vi "worker_loop.vi"(8 "error in (no error)":errorcluster, 10 "Notifiers":T1, 11 "Message Queues":T2) -> (0 "error out":errorcluster)   [LabVIEW 2017, in "worker.lvlib"]
uses:
  worker.lvlib
  support/Message Queue/All Message Queues.ctl
  support/Message Queue/Message Cluster.ctl
  support/Notifiers/Notifiers.ctl
  support/my_global.vi
  <vilib>/Utility/error.llb/Error Cluster From Error Code.vi
  <vilib>/ErrorRing/Error Ring.xnode
  support/Message Queue/Message Queue.lvlib
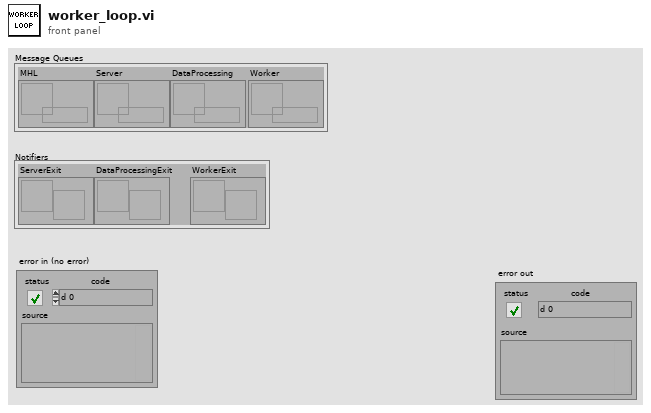
[diagram p1: front panel]
types:
  T1 = typedef "Notifiers.ctl" = cluster{"ServerExit":refnum<notifier>, "DataProcessingExit":refnum<notifier>, "WorkerExit":refnum<notifier>}
  T2 = typedef "Message Queue.lvlib/All Message Queues.ctl" = cluster{"MHL":refnum<queue>, "Server":refnum<queue>, "DataProcessing":refnum<queue>, "Worker":refnum<queue>}
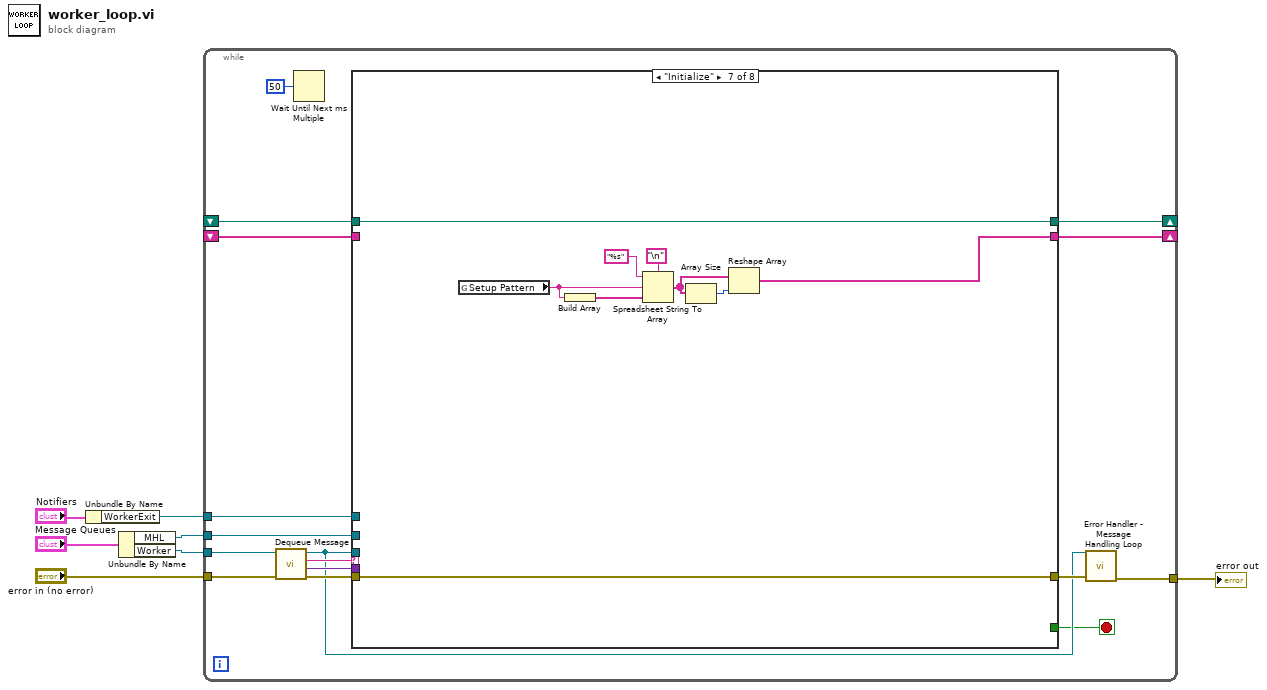
[diagram p0: block diagram]
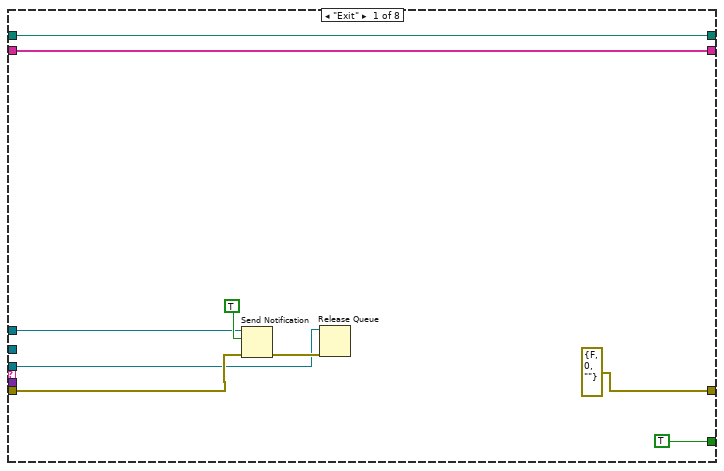
[diagram p2: hidden frame]
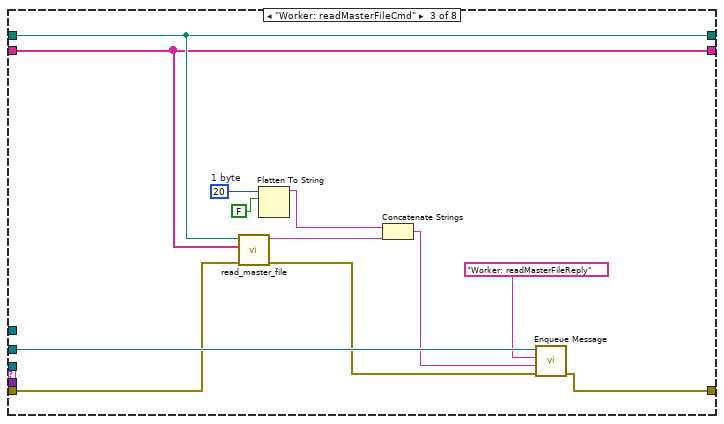
[diagram p4: hidden frame]
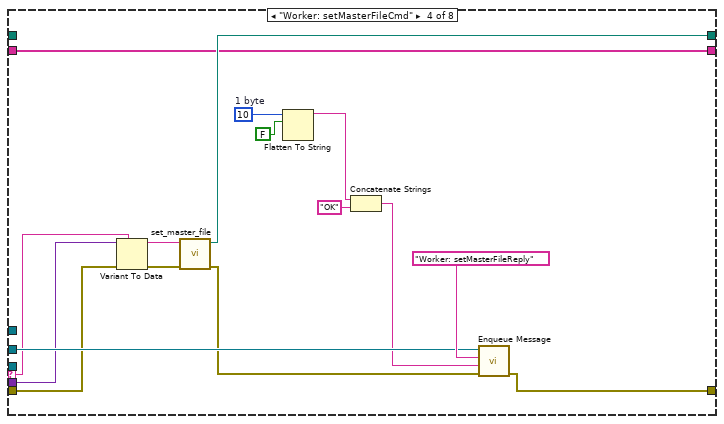
[diagram p5: hidden frame]
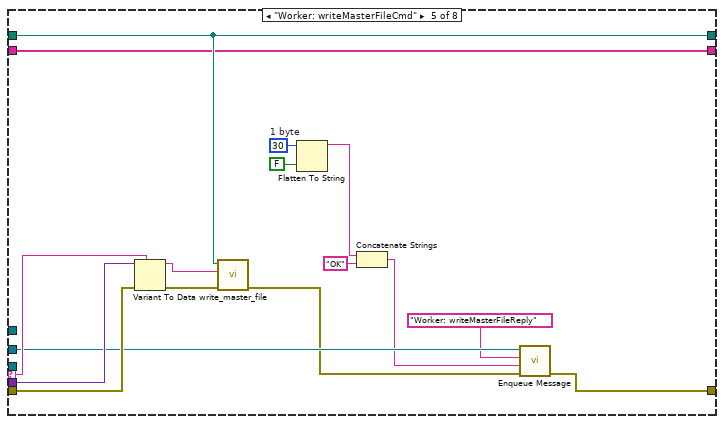
[diagram p6: hidden frame]
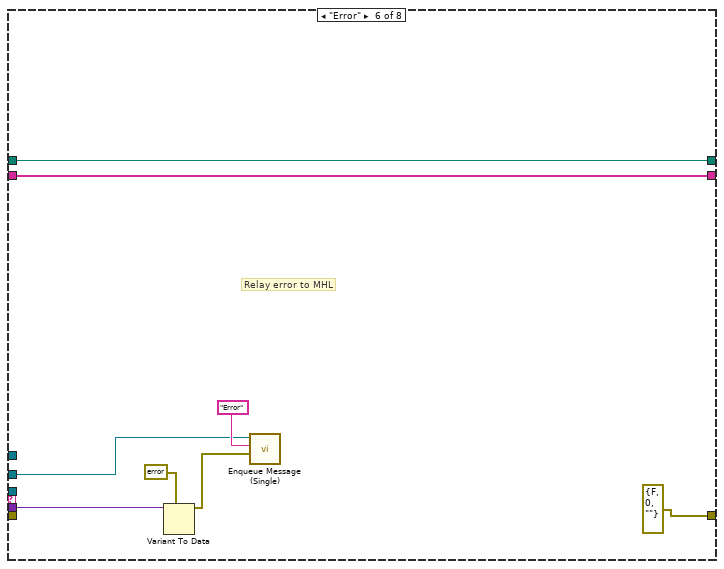
[diagram p7: hidden frame]
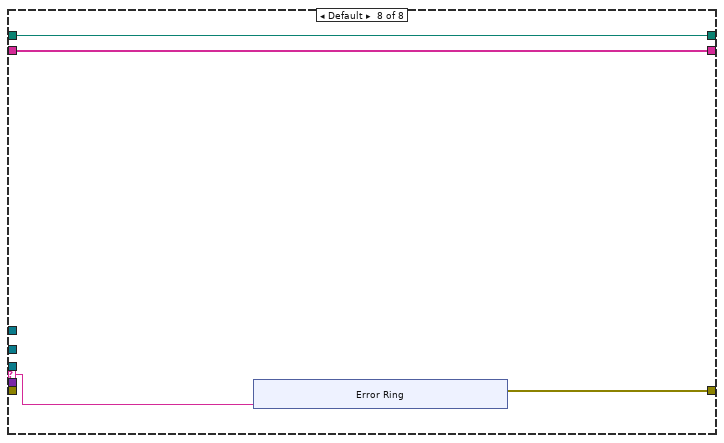
[diagram p8: hidden frame]
diagram:
  n1 = Unbundle By Name("Notifiers") -> ("WorkerExit"=w3:refnum<notifier>)
  n2 = Unbundle By Name("Message Queues") -> ("MHL"=w6:refnum<queue>, "Worker"=w5:refnum<queue>)
  n3 = while {
    tunnel: w6 -> [w17]
    tunnel: w5 -> [w22]
    tunnel: w3 -> [w12]
    tunnel: "error in (no error)" -> [w21]
    tunnel: [w14] -> w1
    shift-right: [w11] -> _
    shift-left: _ -> [w10]
    shift-right: [w9] -> _
    shift-left: _ -> [w8]
    stop <- w13 stop-if-true
    n4 = call "Dequeue Message.vi"("error in (no error)"=w21, "Message Queue"=w22) -> ("error out"=w18:errorcluster, "Message Data"=w19:variant, "Message"=w20:string, "dup Message Queue"=w15:refnum<queue>)  [unwired: 6 in]
    n5 = Wait Until Next ms Multiple(millisecond multiple=u32 50) -> ()  [unwired: 1 out]
    n6 = case shown="\"Initialize\"" w20 {
      selector: w20 -> [_ _ _ w56 w78 _ _ w100]
      tunnel: w15 -> [w28 _ _ _ _ _ _ _]
      tunnel: w19 -> [_ _ _ w55 w79 w83 _ _]
      tunnel: w18 -> [w29 w35 w38 w54 w77 _ w96 _]
      tunnel: w17 -> [_ _ w47 w61 w75 w82 _ _]
      tunnel: [errorcluster {"status"=FALSE, "code"=0, "source"=""} ("error constant") w35 w46 w62 w76 errorcluster {"status"=FALSE, "code"=0, "source"=""} ("error constant") w96 w99] -> w16
      tunnel: [TRUE _ _ _ _ _ _ _] -> w13
      tunnel: w12 -> [w27 _ _ _ _ _ _ _]
      tunnel: [w25 w34 w37 w49 w66 w81 w95 w98] -> w11
      tunnel: w10 -> [w25 w34 w37 _ w66 w81 w95 w98]
      tunnel: [w24 w33 w36 w48 w65 w80 w88 w97] -> w9
      tunnel: w8 -> [w24 w33 w36 w48 w65 w80 _ w97]
      frame "Exit" {
        n7 = Send Notification(notification=TRUE, notifier=w27, error in (no error)=w29) -> (error out=w30:errorcluster)  [unwired: 1 out]
        n8 = Release Queue(queue=w28, error in (no error)=w30) -> ()  [unwired: 1 in, 3 out]
      }
      frame "--- Copy me ---" {
      }
      frame "Worker: readMasterFileCmd" {
        w44 = u8 20  # 1 byte
        n9 = call "read_master_file.vi"("error in (no error)"=w38, "setup file pattern"=w36, "master file path"=w37) -> ("error out"=w42:errorcluster, "setup file paths"=w41:string)  [unwired: 7 in]
        n10 = Flatten To String(anything=w44, prepend array or string size? (T)=FALSE) -> (data string=w40:string)  [unwired: 2 in, 2 out]
        n11 = Concatenate Strings(w40, w41) -> (w39:string)
        n12 = call-poly "Enqueue Message.vi"("error in (no error)"=w42, "Message Data"=w39, "Message"="Worker: readMasterFileReply", "Message Queue"=w47) -> ("error out"=w46:errorcluster)  [unwired: 6 in, 1 out]
      }
      frame "Worker: setMasterFileCmd" {
        w60 = u8 10  # 1 byte
        n13 = Variant To Data(error in=w54, type=w56, Variant=w55) -> (data=w52:string, error out=w53:errorcluster)
        n14 = call "set_master_file.vi"("error in (no error)"=w53, "master file path"=w52) -> ("error out"=w50:errorcluster, "master file path"=w49:path)  [unwired: 8 in]
        n15 = Flatten To String(anything=w60, prepend array or string size? (T)=FALSE) -> (data string=w58:string)  [unwired: 2 in, 2 out]
        n16 = Concatenate Strings(w58, "OK" ("string")) -> (w57:string)
        n17 = call-poly "Enqueue Message.vi"("error in (no error)"=w50, "Message Data"=w57, "Message"="Worker: setMasterFileReply", "Message Queue"=w61) -> ("error out"=w62:errorcluster)  [unwired: 6 in, 1 out]
      }
      frame "Worker: writeMasterFileCmd" {
        w72 = u8 30  # 1 byte
        n18 = Variant To Data(error in=w77, type=w78, Variant=w79) -> (data=w64:string, error out=w74:errorcluster)
        n19 = call "write_master_file.vi"("error in (no error)"=w74, "setup file paths"=w64, "master file path"=w66) -> ("error out"=w73:errorcluster)  [unwired: 8 in]
        n20 = Flatten To String(anything=w72, prepend array or string size? (T)=FALSE) -> (data string=w70:string)  [unwired: 2 in, 2 out]
        n21 = Concatenate Strings(w70, "OK" ("string")) -> (w69:string)
        n22 = call-poly "Enqueue Message.vi"("error in (no error)"=w73, "Message Data"=w69, "Message"="Worker: writeMasterFileReply", "Message Queue"=w75) -> ("error out"=w76:errorcluster)  [unwired: 6 in, 1 out]
      }
      frame "Error" {
        # "Relay error to MHL"
        n23 = Variant To Data(type=errorcluster {"status"=FALSE, "code"=0, "source"=""} ("error constant"), Variant=w83) -> (data=w85:errorcluster)  [unwired: 1 in, 1 out]
        n24 = call "Enqueue Message (Single).vi"("Message Data"=w85, "Message"="Error", "Message Queue"=w82) -> ()  [unwired: 7 in, 2 out]
      }
      frame "Initialize" {
        n25 = global read "my_global.vi" "Setup Pattern"() -> (w94:string)
        n26 = Build Array(w94) -> (w93:string[])
        n27 = Spreadsheet String To Array(delimiter (Tab)="\n", format string="%s", spreadsheet string=w94, array type (2D Dbl)=w93) -> (array=w89:string[])
        n28 = Array Size(array=w89) -> (size(s)=w92:i32)
        n29 = Reshape Array(w89, w92) -> (w88:string[])
      }
      frame Default {
        n30 = xnode "Error Ring"("parameter 0"=w100) -> ("error out"=w99:errorcluster)
      }
    }
    n31 = call "Error Handler - Message Handling Loop.vi"("error in (no error)"=w16, "Message Queue"=w15) -> ("dup error in"=w14:errorcluster)  [unwired: 8 in, 1 out]
  }
  "error out" <- w1
